vi "Add Certificate Paths.vi"(10 "Connection Configuration in":T2) -> (2 "Connection Configuration out":T2)   [LabVIEW 2013, in "OPC UA Server tests.lvlib"]
doc: "Add Certificate paths to module configuration"
uses:
  OPC UA Server tests.lvlib
  <vilib>/OPCUA/server/subVI/supported security policies.ctl
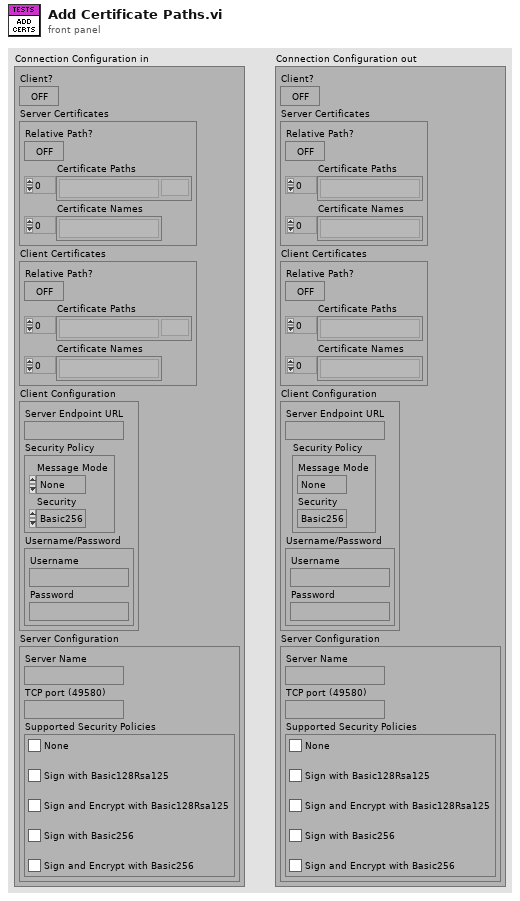
[diagram p1: front panel]
types:
  T1 = typedef "supported security policies.ctl" = cluster{"None":bool, "Sign with Basic128Rsa125":bool, "Sign and Encrypt with Basic128Rsa125":bool, "Sign with Basic256":bool, "Sign and Encrypt with Basic256":bool}
  T2 = cluster{"Client?":bool, "Server Certificates":cluster{"Relative Path?":bool, "Certificate Paths":path[], "Certificate Names":string[]}, "Client Certificates":cluster{"Relative Path?":bool, "Certificate Paths":path[], "Certificate Names":string[]}, "Client Configuration":cluster{"Server Endpoint URL":string, "Security Policy":cluster{"Message Mode":enum16{"None", "Sign", "Sign and Encrypt"}, "Security":enum16{"Basic256", "Basic128Rsa15"}}, "Username/Password":cluster{"Username":string, "Password":string}}, "Server Configuration":cluster{"Server Name":string, "TCP port (49580)":string, "Supported Security Policies":T1}}
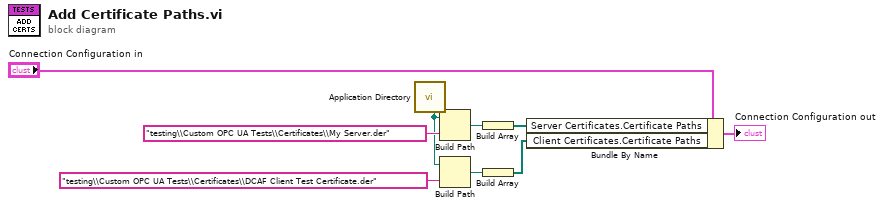
[diagram p0: block diagram]
diagram:
  n1 = call <vilib>:"Application Directory.vi"() -> ("Application Directory"=w2:path)
  n2 = Build Path(base path=w2, name or relative path="testing\\Custom OPC UA Tests\\Certificates\\My Server.der") -> (appended path=w6:path)
  n3 = Build Path(base path=w2, name or relative path="testing\\Custom OPC UA Tests\\Certificates\\DCAF Client Test Certificate.der") -> (appended path=w8:path)
  n4 = Build Array(w6) -> (w7:path[])
  n5 = Build Array(w8) -> (w9:path[])
  n6 = Bundle By Name(cluster="Connection Configuration in", "Server Certificates.Certificate Paths"=w7, "Client Certificates.Certificate Paths"=w9) -> (→"Connection Configuration out":T2)
